vi "ReleaseDbServer.vi"(0 "DashboardServer in":refnum<class "Dashboard Server.lvclass">, 5 "error in (no error)":errorcluster) -> (14 "DashboardServer out":refnum<class "Dashboard Server.lvclass">, 19 "error out":errorcluster)   [LabVIEW 2019, in "Dashboard Server.lvclass"]
uses:
  Dashboard Server.lvclass
  Dashboard Server.lvclass/Dashboard Server.ctl
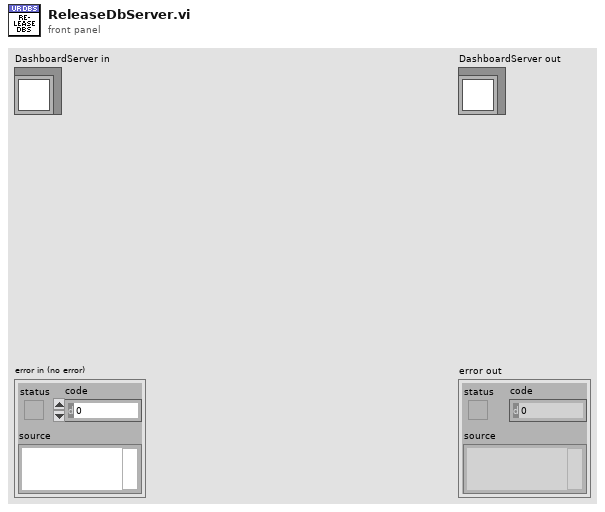
[diagram p1: front panel]
types:
  T1 = typedef "Semaphore RefNum" = refnum<k1>
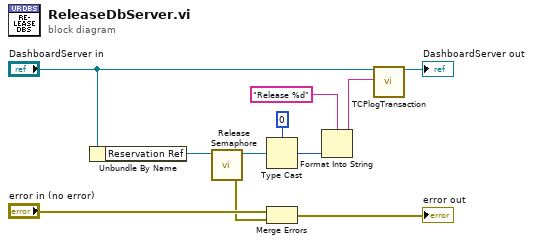
[diagram p0: block diagram]
diagram:
  n1 = Unbundle By Name("DashboardServer in") -> ("Reservation Ref"=w11:T1)
  n2 = call <vilib>:"Release Semaphore.vi"("semaphore"=w11) -> ("error out"=w8:errorcluster, "semaphore out"=w5:T1)  [unwired: 5 in]
  n3 = Type Cast(type=0, x=w5) -> (*(type *) &x=w6:i32)
  n4 = Merge Errors("error in (no error)", w8) -> (→"error out":errorcluster)
  n5 = Format Into String(format string="Release %d", w6) -> (resulting string=w2:string)  [unwired: 2 in, 1 out]
  n6 = call "TCPlogTransaction.vi"("Dashboard Server in"="DashboardServer in", "Transaction"=w2) -> ("Dashboard Server out"=→"DashboardServer out":refnum<class "Dashboard Server.lvclass">)  [unwired: 17 in]
